vi "Read Timer Direction.vi"(8 "error in (no error)":errorcluster, 11 "TimerSensorConfig in":refnum<class "TimerSensorConfig.lvclass">) -> (0 "error out":errorcluster, 2 "Timer Direction":T1, 3 "TimerSensorConfig out":refnum<class "TimerSensorConfig.lvclass">)   [LabVIEW 2012, in "TimerSensor.lvlib" / "TimerSensorConfig.lvclass"]
uses:
  TimerSensorConfig.lvclass
  TimerView Sensor/Timer Direction.ctl
  TimerSensorConfig.lvclass/TimerSensorConfig.ctl
  TimerSensor.lvlib
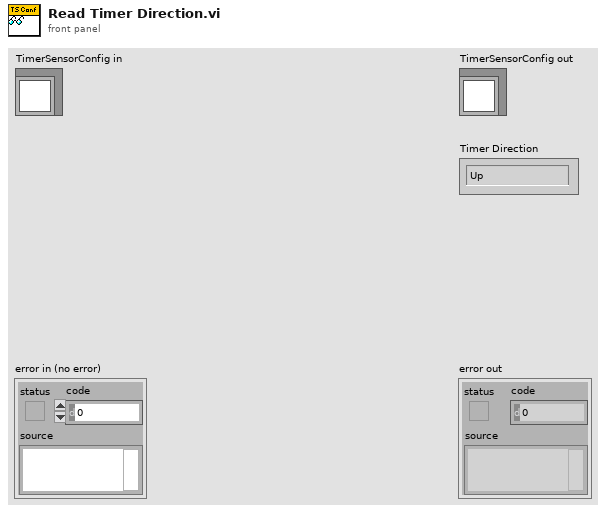
[diagram p1: front panel]
types:
  T1 = typedef "TimerSensor.lvlib/Timer Direction.ctl" = enum16{"Up", "Down"}
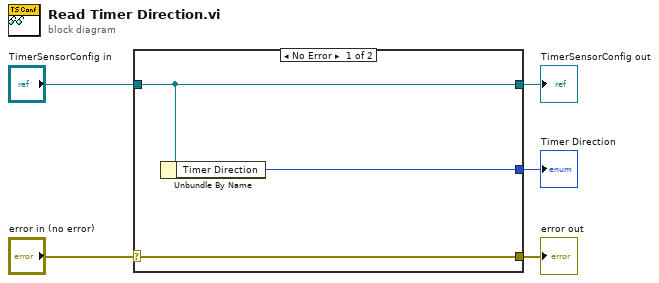
[diagram p0: block diagram]
diagram:
  n1 = case shown="No Error" "error in (no error)" {
    selector: "error in (no error)" -> [w8 w9]
    tunnel: [w8 w9] -> w4
    tunnel: [w7 w10] -> w2
    tunnel: "TimerSensorConfig in" -> [w7 w10]
    tunnel: [w6 _] -> w1
    frame No Error {
      n2 = Unbundle By Name(w7) -> ("Timer Direction"=w6:T1)
    }
    frame Error {
    }
  }
  "error out" <- w4
  "TimerSensorConfig out" <- w2
  "Timer Direction" <- w1
